vi "WLC fit get residue.vi"(4 "control Cluster":T1={"laser power (mW)"=10.0, "center position shift (um)"=0.0001, "center QPD shift (V)"=0.0001, "Fc-cal-array"=[0.004414, 0.00367], "Convf-cal-array"=[0.19240621, 0.01244886], "Length offset"=400.0, "Force offset"=4.0, "trap height(nm)"=300.0, "bead radius(nm)"=515.0, "xDNA cut outside (nm)"=2000.0, "initial parameters"=[40.0, 1150.0], "fit only one side?"=FALSE, "T=positive (RHS)\nF=negative (LHS)"=FALSE, "Position Array Out"=[], "QPD signal Out"=[], "ci"=0.0, "yi"=0.0, "cr"=0.0, "yr"=0.0, "Force constant (pN/nm)"=0.0154, "conversion factor (V/um)"=2.6, "best fit parameters"=[], "best nonlinear fit"=[], "residue"=0.0, "Force-cut 2"=[], "xDNA-cut 2"=[]}) -> (1 "output cluster":T1={"laser power (mW)"=10.0, "center position shift (um)"=0.0001, "center QPD shift (V)"=0.0001, "Fc-cal-array"=[0.004414, 0.00367], "Convf-cal-array"=[0.19240621, 0.01244886], "Length offset"=400.0, "Force offset"=4.0, "trap height(nm)"=300.0, "bead radius(nm)"=515.0, "xDNA cut outside (nm)"=2000.0, "initial parameters"=[40.0, 1150.0], "fit only one side?"=FALSE, "T=positive (RHS)\nF=negative (LHS)"=FALSE, "Position Array Out"=[], "QPD signal Out"=[], "ci"=0.0, "yi"=0.0, "cr"=0.0, "yr"=0.0, "Force constant (pN/nm)"=0.0154, "conversion factor (V/um)"=2.6, "best fit parameters"=[], "best nonlinear fit"=[], "residue"=0.0, "Force-cut 2"=[], "xDNA-cut 2"=[]})   [LabVIEW 2014]
uses:
  Control cluster.ctl
  <vilib>/gmath/NumericalOptimization/Nonlinear Curve Fit LM formula string.vi
  <vilib>/gmath/NI_Gmath.lvlib
panel:
  # "Lp"
  # "L0"
  # "Lp"
  # "L0"
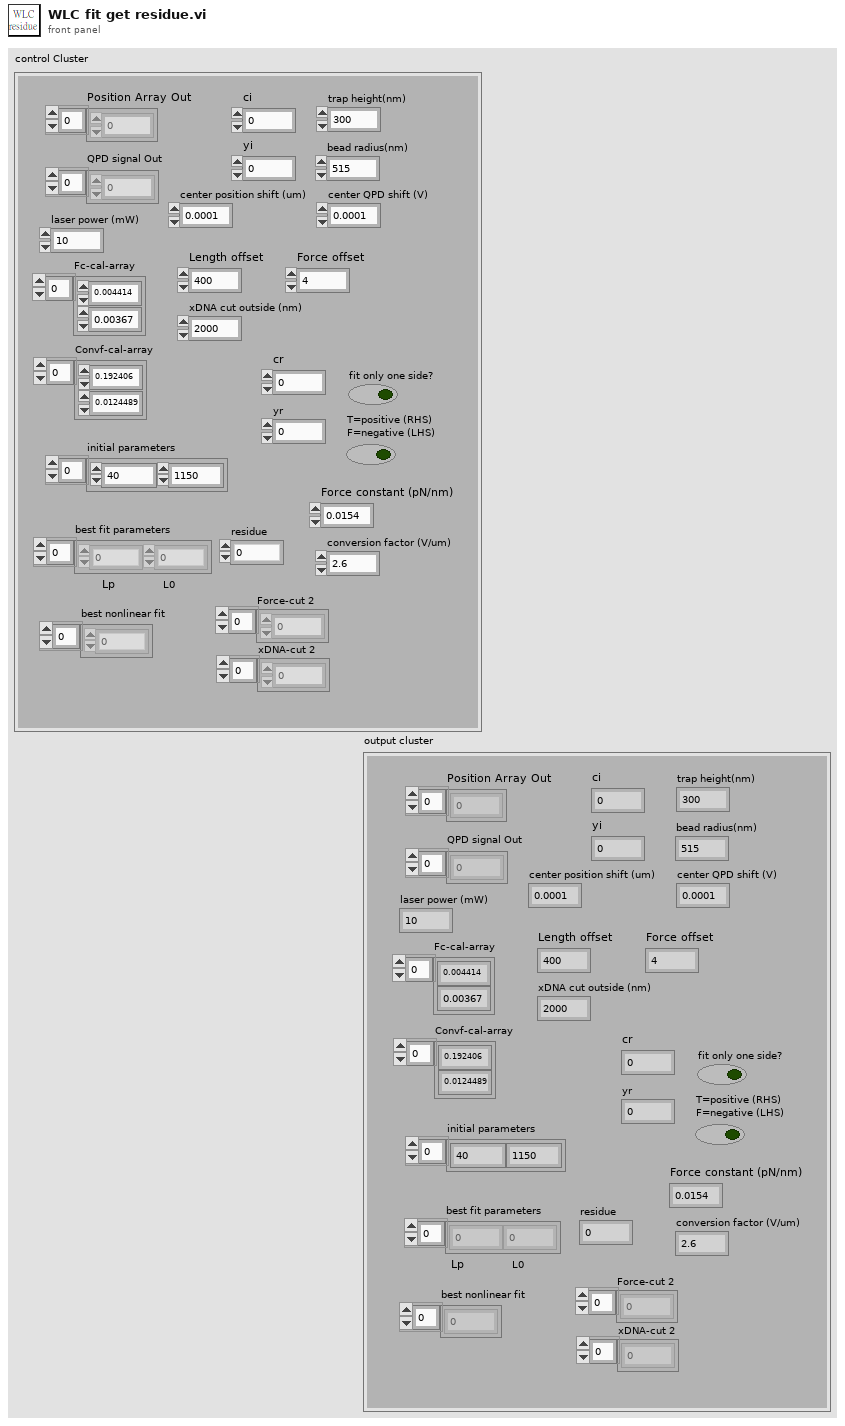
[diagram p1: front panel]
types:
  T1 = typedef "Control cluster.ctl" = cluster{"laser power (mW)":dbl, "center position shift (um)":dbl, "center QPD shift (V)":dbl, "Fc-cal-array":dbl[], "Convf-cal-array":dbl[], "Length offset":dbl, "Force offset":dbl, "trap height(nm)":dbl, "bead radius(nm)":dbl, "xDNA cut outside (nm)":dbl, "initial parameters":dbl[], "fit only one side?":bool, "T=positive (RHS)\nF=negative (LHS)":bool, "Position Array Out":dbl[], "QPD signal Out":dbl[], "ci":dbl, "yi":dbl, "cr":dbl, "yr":dbl, "Force constant (pN/nm)":dbl, "conversion factor (V/um)":dbl, "best fit parameters":dbl[], "best nonlinear fit":dbl[], "residue":dbl, "Force-cut 2":dbl[], "xDNA-cut 2":dbl[]}
  T2 = cluster{"model":string, "Parameters":string[], "x":string}
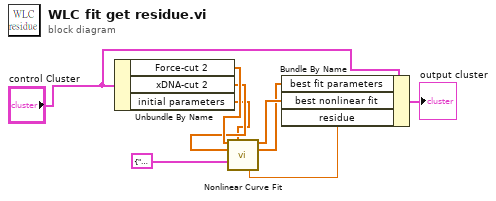
[diagram p0: block diagram]
diagram:
  n1 = Unbundle By Name("control Cluster") -> ("Force-cut 2"=w8:dbl[], "xDNA-cut 2"=w7:dbl[], "initial parameters"=w6:dbl[])
  n2 = call-poly <vilib>:"Nonlinear Curve Fit.vi"("Y"=w8, "initial parameters"=w6, "X"=w7, "model description"=T2 {"model"="4.08687*(1/a1)*(sign(u)*1/4*(1-sign(u)*u/a2)^(-2)-(1/4*sign(u))+u/a2)", "Parameters"=["a1", "a2"], "x"="u"}) -> ("best nonlinear fit"=w4:dbl[], "best fit parameters"=w3:dbl[], "residue"=w2:dbl)  [unwired: 3 in, 6 out]
  n3 = Bundle By Name(cluster="control Cluster", "best fit parameters"=w3, "best nonlinear fit"=w4, "residue"=w2) -> (→"output cluster":T1)
